vi "Configure Filter (Frequency).vi"(7 "Element (0: All)":i32(ring) items=["All", "1", "2", "3", "4", "5", "6"], 8 "error in (no error)":errorcluster, 9 "Cutoff Frequency (100Hz)":i32(ring)=100 items=["100"=100, "1000"=1000], 10 "Enable Frequency Filter (T: Enable)":bool=TRUE, 11 "VISA resource name":refnum<visa-resource-name>) -> (0 "error out":errorcluster, 3 "VISA resource name out":refnum<visa-resource-name>)   [LabVIEW 2021, in "Yokogawa WT1800 Series.lvlib"]
doc: "Configures the frequency filter features."
uses:
  <instrlib>/Yokogawa WT1800 Series/Yokogawa WT1800 Series.lvlib
panel:
  # "Hz"
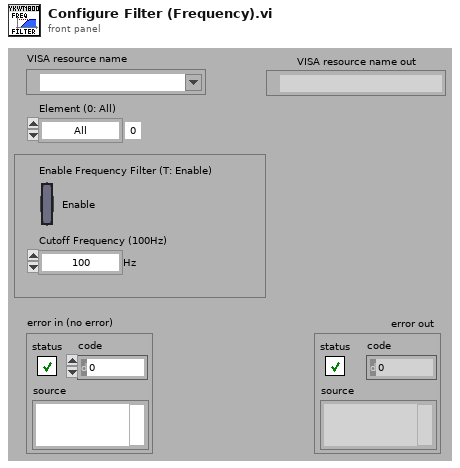
[diagram p1: front panel]
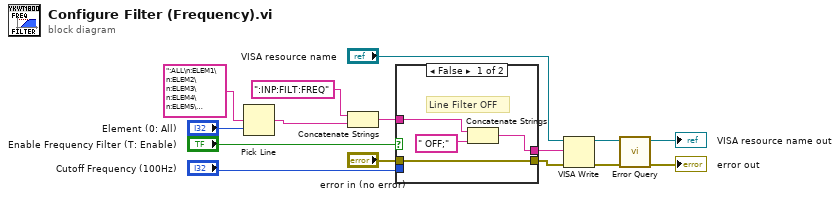
[diagram p0: block diagram]
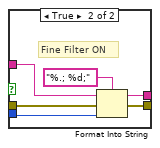
[diagram p2: hidden frame]
diagram:
  n1 = Pick Line ("ライン選択")(multi-line string=":ALL\n:ELEM1\n:ELEM2\n:ELEM3\n:ELEM4\n:ELEM5\n:ELEM6\n:SIGMA\n:SIGMB\n:SIGMC" ("複数行文字列"), line index="Element (0: All)") -> (output string=w7:string)  [unwired: 1 in]
  n2 = Concatenate Strings(":INP:FILT:FREQ", w7) -> (w6:string)
  n3 = case "ケースストラクチャ" shown="False" "Enable Frequency Filter (T: Enable)" {
    tunnel: w6 -> [w18 w24]
    tunnel: "error in (no error)" -> [w16 w23]
    tunnel: [w17 w22] -> w3
    tunnel: [w16 w21] -> w2
    tunnel: "Cutoff Frequency (100Hz)" -> [_ w20]
    frame False {
      # "Line Filter OFF"
      n4 = Concatenate Strings(w18, " OFF;" ("文字列")) -> (w17:string)
    }
    frame True {
      # "Fine Filter ON"
      n5 = Format Into String ("文字列にフォーマット")(format string="%.; %d;" ("形式文字列"), initial string=w24, error in=w23, w20) -> (resulting string=w22:string, error out=w21:errorcluster)
    }
  }
  n6 = VISA Write ("VISA書き込み")(VISA resource name="VISA resource name", write buffer=w3, error in (no error)=w2) -> (VISA resource name out=w15:refnum<visa-resource-name>, error out=w14:errorcluster)  [unwired: 1 out]
  n7 = call <instrlib>:"Error Query.vi"("error in (no error)"=w14, "VISA resource name"=w15) -> ("error out"=→"error out":errorcluster, "VISA resource name out"=→"VISA resource name out":refnum<visa-resource-name>)  [unwired: 6 in, 2 out]
